vi "Initialize REF Channels.vi"(8 "error in (no error)":errorcluster, 11 "Instrument.Lockin":refnum<class "Instrument.Lockin.lvclass">) -> (0 "error out":errorcluster, 3 "Instrument.Lockin out":refnum<class "Instrument.Lockin.lvclass">)   [LabVIEW 2016, in "Instrument.Lockin.lvclass"]
uses:
  Instrument.Lockin.lvclass
  LockinDAQ/Typedefs/REF-cluster.ctl
  LockinDAQ/LockinDAQ.lvclass
panel:
  out "cluster out":T1={"Ch"=[13], " f (Hz)"=[13.0], "Phase (°)"=[0.0], "TC (s)"=[0.0001, 0.0001, 0.0001, 0.0001], "order"=[0]} {"order" min=1; "TC (s)" min=0.0001 format="%#_3p"; "Phase (°)" format="%.3g"; "f (Hz)" format="%.3g"}
  out "cluster in":T1={"Ch"=[13], " f (Hz)"=[13.0], "Phase (°)"=[0.0], "TC (s)"=[0.0001, 0.0001, 0.0001, 0.0001], "order"=[0]} {"order" min=1; "TC (s)" min=0.0001 format="%#_3p"; "Phase (°)" format="%.3g"; "f (Hz)" format="%.3g"}
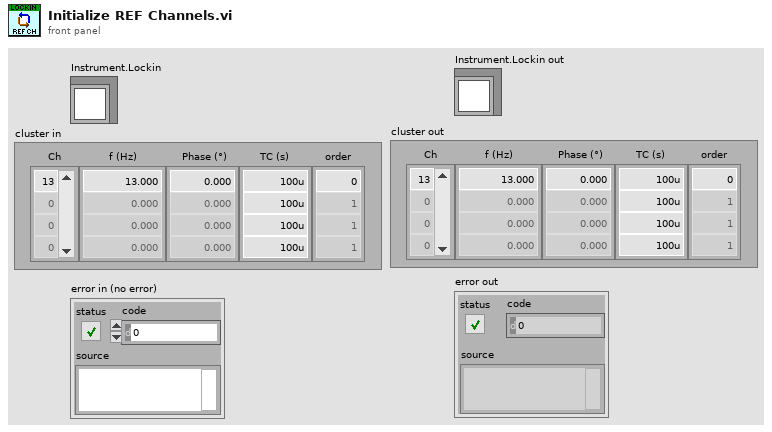
[diagram p1: front panel]
types:
  T1 = typedef "LockinDAQ.lvclass/REF-cluster.ctl" = cluster{"Ch":i32[], " f (Hz)":dbl[], "Phase (°)":dbl[], "TC (s)":dbl[], "order":i32[]}
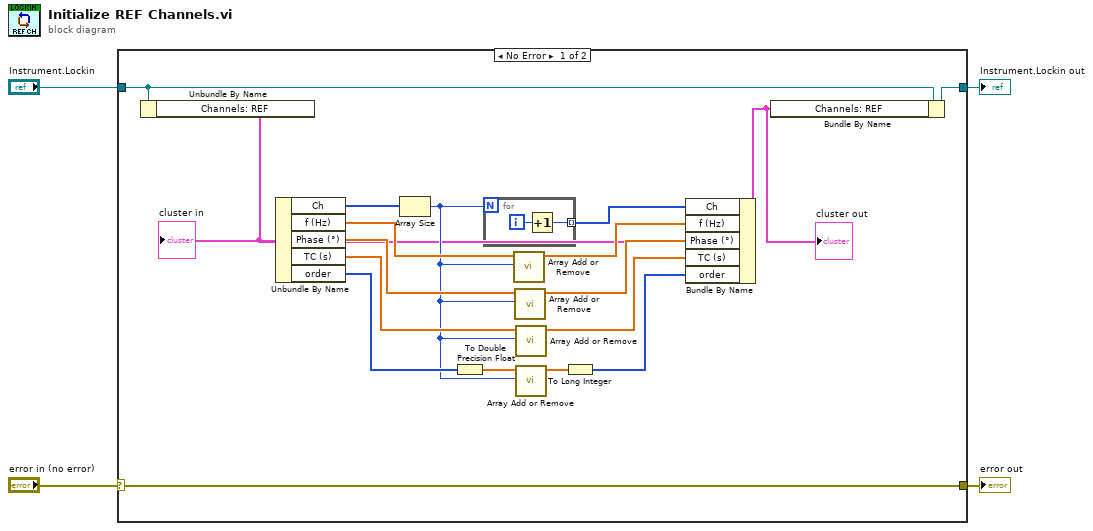
[diagram p0: block diagram]
diagram:
  n1 = case shown="No Error" "error in (no error)" {
    selector: "error in (no error)" -> [w20 w26]
    tunnel: "Instrument.Lockin" -> [w19 w25]
    tunnel: [w21 w25] -> w3
    tunnel: [w20 w26] -> w1
    frame No Error {
      n2 = Unbundle By Name(w19) -> ("Channels: REF"=w5:T1)
      "cluster in" <- w5
      n3 = Unbundle By Name(w5) -> ("Ch"=w22:i32[], "f (Hz)"=w16:dbl[], "Phase (°)"=w15:dbl[], "TC (s)"=w14:dbl[], "order"=w13:i32[])
      n4 = Array Size(array=w22) -> (size(s)=w9:i32)
      n5 = To Double Precision Float(number=w13) -> (double precision float=w7:dbl[])
      n6 = for {
        N: w9 -> [_]
        tunnel: [w23] -> w8 mode=indexing
        i -> [w24]
        n7 = Increment(x=w24) -> (x+1=w23:i32)
      }
      n8 = call "Array Add or Remove.vi"("Size"=w9, "Array in"=w16) -> ("Arry out"=w17:dbl[])  [unwired: 9 in]
      n9 = call "Array Add or Remove.vi"("Size"=w9, "Array in"=w15) -> ("Arry out"=w12:dbl[])  [unwired: 9 in]
      n10 = call "Array Add or Remove.vi"("Size"=w9, "Array in"=w14) -> ("Arry out"=w11:dbl[])  [unwired: 9 in]
      n11 = call "Array Add or Remove.vi"("Size"=w9, "Array in"=w7) -> ("Arry out"=w10:dbl[])  [unwired: 9 in]
      n12 = To Long Integer(number=w10) -> (32bit integer=w6:i32[])
      n13 = Bundle By Name(cluster=w5, "Ch"=w8, "f (Hz)"=w17, "Phase (°)"=w12, "TC (s)"=w11, "order"=w6) -> (w18:T1)
      "cluster out" <- w18
      n14 = Bundle By Name(cluster=w19, "Channels: REF"=w18) -> (w21:refnum<class "Instrument.Lockin.lvclass">)
    }
    frame Error {
    }
  }
  "Instrument.Lockin out" <- w3
  "error out" <- w1
